vi "试剂容量读取.vi"(8 "Error in":errorcluster caption="Error in (no error)", 11 "MB session in":refnum<class "MB_Master.lvclass">) -> (0 "error out":errorcluster, 2 "试剂容量":T1, 3 "MB session out":refnum<class "MB_Master.lvclass">)   [LabVIEW 2016, in "斯坦道总氮.lvlib"]
uses:
  <vilib>/Plasmionique/MB Master/MB_Master/MB_Master.lvclass
  <vilib>/Plasmionique/MB Master/MB Master.lvlib
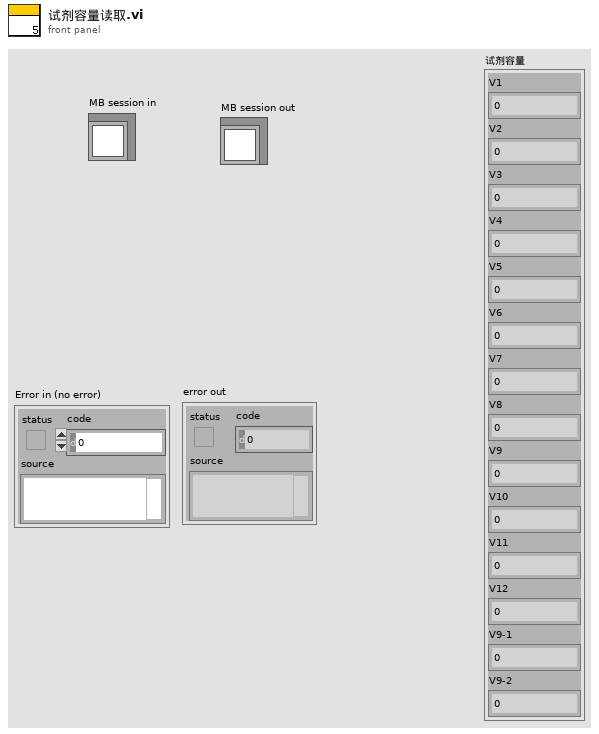
[diagram p1: front panel]
types:
  T1 = cluster{"V1":u16, "V2":u16, "V3":u16, "V4":u16, "V5":u16, "V6":u16, "V7":u16, "V8":u16, "V9":u16, "V10":u16, "V11":u16, "V12":u16, "V9-1":u16, "V9-2":u16}
  T2 = cluster{"WORD[0]":u16, "WORD[1]":u16, "WORD[2]":u16, "WORD[3]":u16, "WORD[4]":u16, "WORD[5]":u16, "WORD[6]":u16, "WORD[7]":u16, "WORD[8]":u16, "WORD[9]":u16, "WORD[10]":u16, "WORD[11]":u16, "WORD[12]":u16, "WORD[13]":u16}
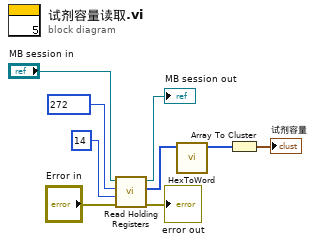
[diagram p0: block diagram]
diagram:
  n1 = call <vilib>:"Read Holding Registers.vi"("error in (no error)"="Error in", "quantity"=u16 14, "starting address"=u16 272, "MB session in"="MB session in") -> ("error out"=→"error out":errorcluster, "Registers"=w2:u16[], "MB session out"=→"MB session out":refnum<class "MB_Master.lvclass">)  [unwired: 5 in]
  n2 = call "HexToWord.vi"("数组"=w2) -> ("WORD"=w1:u16[])  [unwired: 10 in]
  n3 = Array To Cluster(array=w1) -> (cluster=→"试剂容量":T2)
